vi "Backup.Code.vi"() -> ()   [LabVIEW 2014]
panel:
  out "Terminal":string
  in  "Stop Button":bool
  in  "Pause Button":bool
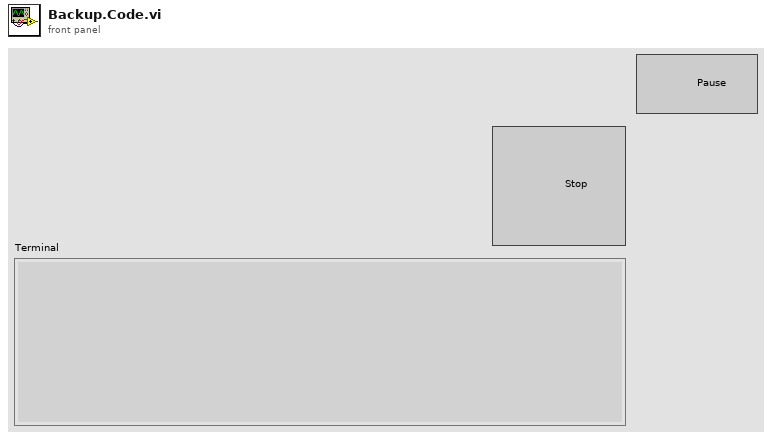
[diagram p1: front panel]
types:
  T1 = typedef "Sensor Reading.ctl" = cluster{"Sensor Name":string, "Time Stamp":timestamp, "Data Chunk":string, "Fractional Time":u64}
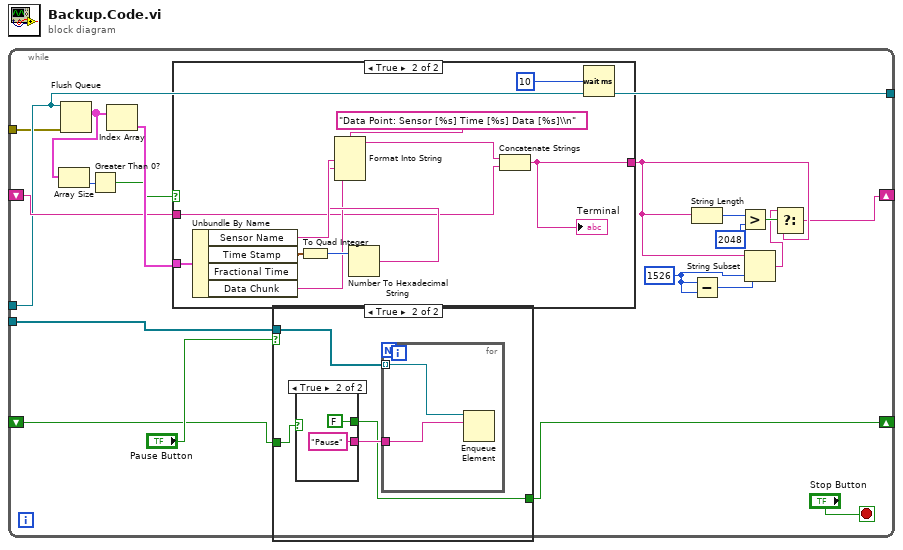
[diagram p0: block diagram]
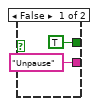
[diagram p3: hidden frame]
diagram:
  n1 = while {
    shift-right: [w6] -> _
    shift-left: [w20] -> w1
    tunnel: _ -> [w19]
    tunnel: [w19] -> _
    tunnel: _ -> [w18]
    tunnel: _ -> [w5]
    shift-right: [w2] -> _
    shift-left: _ -> [w3]
    stop <- "Stop Button" stop-if-true
    w8 = 1526 ("y")
    n2 = Flush Queue(queue=w19, error in (no error)=w18) -> (remaining elements=w15:T1[])  [unwired: 2 out]
    n3 = Array Size(array=w15) -> (size(s)=w16:i32)
    n4 = Greater Than 0?(x=w16) -> (x > 0?=w14:bool)
    n5 = Index Array(array=w15) -> (element=w21:T1)  [unwired: 1 in]
    n6 = case shown="True" w14 {
      tunnel: w21 -> [_ w42]
      tunnel: w20 -> [w33 w35]
      tunnel: [w33 w34] -> w7
      frame False {
      }
      frame True {
        n7 = Unbundle By Name(w42) -> ("Sensor Name"=w41:string, "Time Stamp"=w40:timestamp, "Data Chunk"=w37:string)  [unwired: 1 out]
        n8 = To Quad Integer(1:w40) -> (0:w39:i64)
        n9 = Number To Hexadecimal String(2:w39) -> (0:w38:string)  [unwired: 1 in]
        n10 = Format Into String(format string="Data Point: Sensor [%s] Time [%s] Data [%s]\\n", w41, w38, w37) -> (resulting string=w36:string)  [unwired: 2 in, 1 out]
        n11 = Concatenate Strings(w36, w35) -> (w34:string)
        "Terminal" <- w34
        n12 = Wait (ms)(milliseconds to wait=u32 10) -> ()  [unwired: 1 out]
      }
    }
    n13 = case shown="True" "Pause Button" {
      tunnel: w5 -> [_ w26]
      tunnel: w3 -> [w22 w24]
      tunnel: [w22 w23] -> w2
      frame False {
      }
      frame True {
        n14 = case shown="True" w24 {
          tunnel: ["Unpause" ("element") "Pause" ("element")] -> w25
          tunnel: [TRUE FALSE] -> w23
          frame False {
          }
          frame True {
          }
        }
        n15 = for {
          tunnel: w26 -> [w32] mode=indexing
          tunnel: w25 -> [w31]
          n16 = Enqueue Element(queue=w32, element=w31) -> ()  [unwired: 2 in, 3 out]
        }
      }
    }
    n17 = String Length(string=w7) -> (length=w10:i32)
    n18 = Subtract(x=w8, y=w8) -> (x-y=w11:i32)
    n19 = Greater?(x=w10, y=2048) -> (0:w12:bool)
    n20 = String Subset(string=w7, offset (0)=w11, length (rest)=w8) -> (substring=w9:string)
    n21 = Select(t=w9, s=w12, f=w7) -> (s? t:f=w6:string)
  }
